vi "ARC_Dynamic Call_Reentrant.vi"(5 "command queue name":string, 6 "time out(5s)":dbl=5.0, 7 "open front panel? (T)":bool=TRUE, 8 "error in (no error)":errorcluster, 9 "parameter else":variant, 10 "control name":string, 11 "vi path":path) -> (0 "error out":errorcluster, 1 "time out":bool, 2 "call failed":bool, 3 "VI Ref":refnum<vi>)   [LabVIEW 2016]
uses:
  Queue Management/ARC_Queue Valid.vi
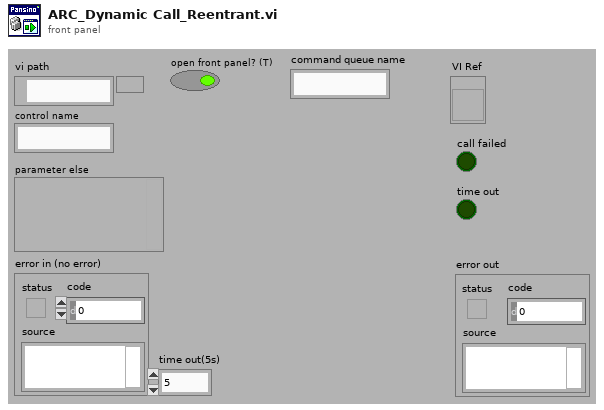
[diagram p1: front panel]
types:
  T1 = enum32{"Invalid", "Standard", "Closed", "Hidden", "Minimized", "Maximized"}
  T2 = cluster{"command queue name":string, "parameter else":variant}
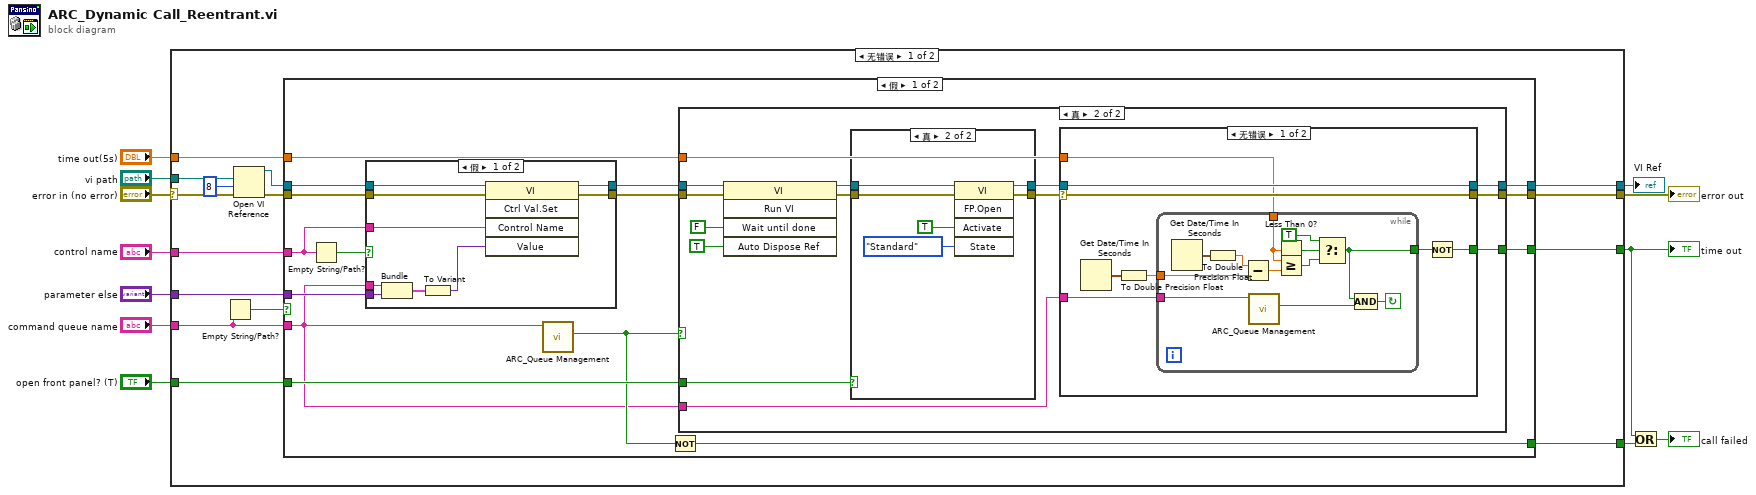
[diagram p0: block diagram]
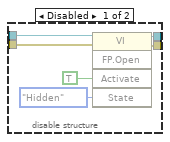
[diagram p5: hidden frame]
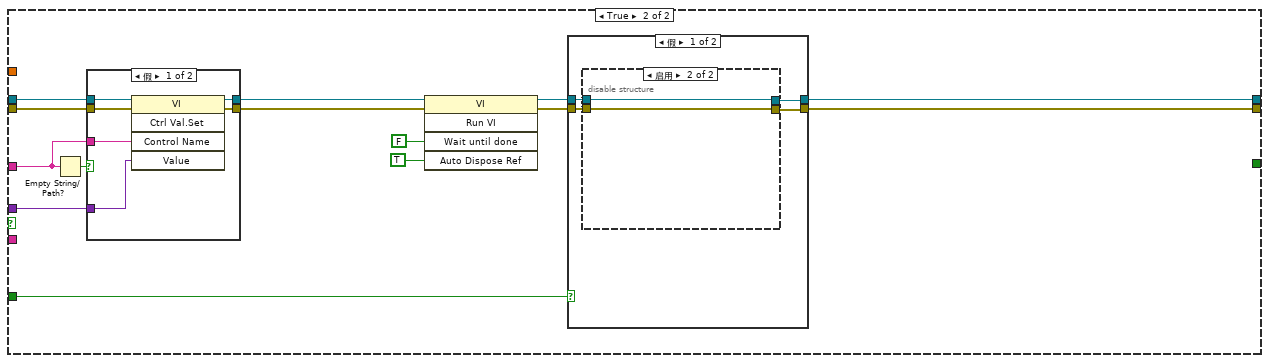
[diagram p7: hidden frame]
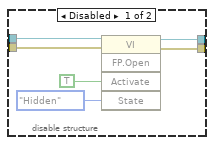
[diagram p9: hidden frame]
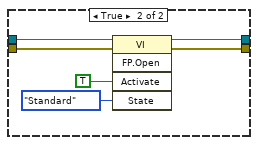
[diagram p10: hidden frame]
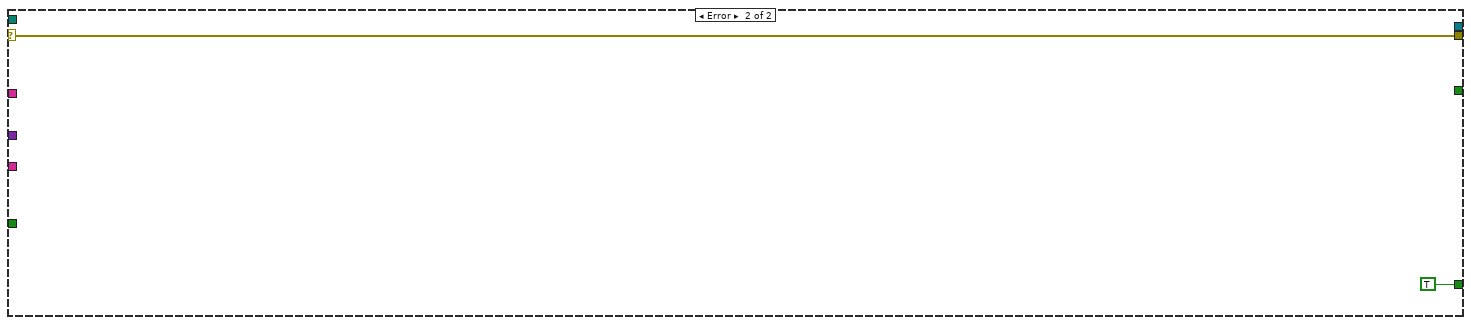
[diagram p11: hidden frame]
diagram:
  n1 = case shown="无错误" "error in (no error)" {
    selector: "error in (no error)" -> [w27 w151]
    tunnel: [w17 w151] -> w11
    tunnel: "vi path" -> [w26 _]
    tunnel: "open front panel? (T)" -> [w25 _]
    tunnel: "control name" -> [w24 _]
    tunnel: "command queue name" -> [w23 _]
    tunnel: "parameter else" -> [w22 _]
    tunnel: "time out(5s)" -> [w21 _]
    tunnel: [w20 TRUE] -> w3
    tunnel: [w19 _] -> w4
    tunnel: [w13 _] -> w1
    frame No Error {
      n2 = Empty String/Path?(string/path=w23) -> (empty?=w16:bool)
      n3 = Open VI Reference(vi path=w26, options=8, error in (no error)=w27) -> (vi reference=w14:refnum<vi>, error out=w15:errorcluster)  [unwired: 3 in]
      n4 = case shown="假" w16 {
        tunnel: [w42 w123] -> w13
        tunnel: [w41 w122] -> w17
        tunnel: w25 -> [w40 w121]
        tunnel: w14 -> [w39 w120]
        tunnel: w15 -> [w38 w119]
        tunnel: w24 -> [w37 w118]
        tunnel: w23 -> [w28 _]
        tunnel: w22 -> [w31 w111]
        tunnel: w21 -> [w35 _]
        tunnel: [w33 _] -> w20
        tunnel: [w32 _] -> w19
        frame False {
          n5 = Empty String/Path?(string/path=w37) -> (empty?=w36:bool)
          n6 = case shown="假" w36 {
            tunnel: w39 -> [w107 w109]
            tunnel: [w106 w109] -> w30
            tunnel: [w105 w108] -> w29
            tunnel: w38 -> [w104 w108]
            tunnel: w37 -> [w103 _]
            tunnel: w31 -> [w101 _]
            tunnel: w28 -> [w102 _]
            frame False {
              n7 = Bundle("command queue name"=w102, "parameter else"=w101) -> (w100:T2)  [unwired: 1 in]
              n8 = To Variant(anything=w100) -> (Variant=w99:variant)
              n9 = invoke class="VI" method="Ctrl Val.Set"(reference=w107, error in=w104, "Control Name"=w103, "Value"=w99) -> (reference out=w106:refnum<vi>, error out=w105:errorcluster)  [unwired: 1 in, 3 out]
            }
            frame True {
            }
          }
          n10 = call-poly "ARC_Queue Management.vi"("Queue Name(unamed)"=w28) -> ("Not Exist?"=w34:bool)  [unwired: 8 in, 2 out]
          n11 = Not(x=w34) -> (.not. x?=w33:bool)
          n12 = case shown="真" w34 {
            tunnel: [w44 w50] -> w42
            tunnel: [w43 w49] -> w41
            tunnel: w40 -> [_ w58]
            tunnel: w30 -> [w44 w55]
            tunnel: w29 -> [w43 w54]
            tunnel: w28 -> [_ w47]
            tunnel: w35 -> [_ w48]
            tunnel: [_ w46] -> w32
            frame False {
            }
            frame True {
              n13 = invoke class="VI" method="Run VI"(reference=w55, error in=w54, "Wait until done"=FALSE, "Auto Dispose Ref"=TRUE ("Auto Dispose Reference")) -> (reference out=w56:refnum<vi>, error out=w57:errorcluster)  [unwired: 1 in, 3 out]
              n14 = case shown="真" w58 {
                tunnel: w57 -> [w82 w94]
                tunnel: w56 -> [w84 w96]
                tunnel: [w83 w95] -> w51
                tunnel: [w81 w93] -> w52
                frame False {
                  n15 = disable-structure shown="启用" {
                    disable-tunnel: w84 -> [w88 w92]
                    disable-tunnel: [w87 w92] -> w83
                    disable-tunnel: w82 -> [w86 w91]
                    disable-tunnel: [w85 w91] -> w81
                    frame Disabled {
                      n16 = invoke class="VI" method="FP.Open"(reference=w88, error in=w86, "Activate"=TRUE ("激活？"), "State"=T1."Hidden" ("状态")) -> (reference out=w87:refnum<vi>, error out=w85:errorcluster)  [unwired: 1 in, 3 out]
                    }
                    frame Enabled {
                    }
                  }
                }
                frame True {
                  n17 = invoke class="VI" method="FP.Open"(reference=w96, error in=w94, "Activate"=TRUE ("激活？"), "State"=T1."Standard" ("状态")) -> (reference out=w95:refnum<vi>, error out=w93:errorcluster)  [unwired: 1 in, 3 out]
                }
              }
              n18 = case shown="无错误" w52 {
                selector: w52 -> [w65 w79]
                tunnel: w51 -> [w66 w80]
                tunnel: [w66 w80] -> w50
                tunnel: [w65 w79] -> w49
                tunnel: w47 -> [w62 _]
                tunnel: w48 -> [w61 _]
                tunnel: [w59 _] -> w46
                frame No Error {
                  n19 = Get Date/Time In Seconds() -> (seconds since 1Jan1904=w63:timestamp)
                  n20 = To Double Precision Float(number=w63) -> (double precision float=w64:dbl)
                  n21 = while {
                    tunnel: w64 -> [w76]
                    tunnel: w62 -> [w71]
                    tunnel: w61 -> [w70]
                    tunnel: [w67] -> w60
                    stop <- w73 continue-if-true
                    n22 = Get Date/Time In Seconds() -> (seconds since 1Jan1904=w77:timestamp)
                    n23 = To Double Precision Float(number=w77) -> (double precision float=w78:dbl)
                    n24 = Subtract(x=w78, y=w76) -> (x-y=w75:dbl)
                    n25 = call-poly "ARC_Queue Management.vi"("Queue Name(unamed)"=w71) -> ("Not Exist?"=w74:bool)  [unwired: 8 in, 2 out]
                    n26 = Less Than 0?(x=w70) -> (x < 0?=w69:bool)
                    n27 = Greater Or Equal?(x=w70, y=w75) -> (x >= y?=w72:bool)
                    n28 = Select(t=TRUE, s=w69, f=w72) -> (s? t:f=w67:bool)
                    n29 = Compound Arithmetic op=AND(w67, w74) -> (w73:bool)
                  }
                  n30 = Not(x=w60) -> (.not. x?=w59:bool)
                }
                frame Error {
                }
              }
            }
          }
        }
        frame True {
          n31 = Empty String/Path?(string/path=w118) -> (empty?=w112:bool)
          n32 = case shown="假" w112 {
            tunnel: w120 -> [w129 w131]
            tunnel: [w128 w131] -> w115
            tunnel: [w127 w130] -> w114
            tunnel: w119 -> [w126 w130]
            tunnel: w118 -> [w125 _]
            tunnel: w111 -> [w124 _]
            frame False {
              n33 = invoke class="VI" method="Ctrl Val.Set"(reference=w129, error in=w126, "Control Name"=w125, "Value"=w124) -> (reference out=w128:refnum<vi>, error out=w127:errorcluster)  [unwired: 1 in, 3 out]
            }
            frame True {
            }
          }
          n34 = invoke class="VI" method="Run VI"(reference=w115, error in=w114, "Wait until done"=FALSE, "Auto Dispose Ref"=TRUE ("Auto Dispose Reference")) -> (reference out=w116:refnum<vi>, error out=w117:errorcluster)  [unwired: 1 in, 3 out]
          n35 = case shown="假" w121 {
            tunnel: w117 -> [w133 w145]
            tunnel: w116 -> [w135 w147]
            tunnel: [w134 w146] -> w123
            tunnel: [w132 w144] -> w122
            frame False {
              n36 = disable-structure shown="启用" {
                disable-tunnel: w135 -> [w139 w143]
                disable-tunnel: [w138 w143] -> w134
                disable-tunnel: w133 -> [w137 w142]
                disable-tunnel: [w136 w142] -> w132
                frame Disabled {
                  n37 = invoke class="VI" method="FP.Open"(reference=w139, error in=w137, "Activate"=TRUE ("激活？"), "State"=T1."Hidden" ("状态")) -> (reference out=w138:refnum<vi>, error out=w136:errorcluster)  [unwired: 1 in, 3 out]
                }
                frame Enabled {
                }
              }
            }
            frame True {
              n38 = invoke class="VI" method="FP.Open"(reference=w147, error in=w145, "Activate"=TRUE ("激活？"), "State"=T1."Standard" ("状态")) -> (reference out=w146:refnum<vi>, error out=w144:errorcluster)  [unwired: 1 in, 3 out]
            }
          }
        }
      }
    }
    frame Error {
    }
  }
  "error out" <- w11
  "time out" <- w4
  "VI Ref" <- w1
  n39 = Or(x=w4, y=w3) -> (x .or. y?=→"call failed":bool)
